vi "lp-server-events.vi"() -> ()   [LabVIEW 2010]
uses:
  socket_type.ctl
  zmq_context.lvclass
  zeromq.lvlib
  zmq_socket.lvclass
panel:
  out "element":string
  out "time (ms)":u32
  in  "stop?":bool
  in  "endpoint":string="tcp://127.0.0.1:5555"
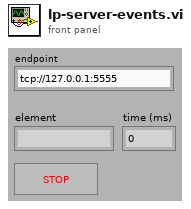
[diagram p1: front panel]
types:
  T1 = typedef "zeromq.lvlib/socket_type.ctl" = enum8{"ZMQ_PAIR", "ZMQ_PUB", "ZMQ_SUB", "ZMQ_REQ", "ZMQ_REP", "ZMQ_DEALER", "ZMQ_ROUTER", "ZMQ_PULL", "ZMQ_PUSH", "ZMQ_XPUB", "ZMQ_XSUB"}
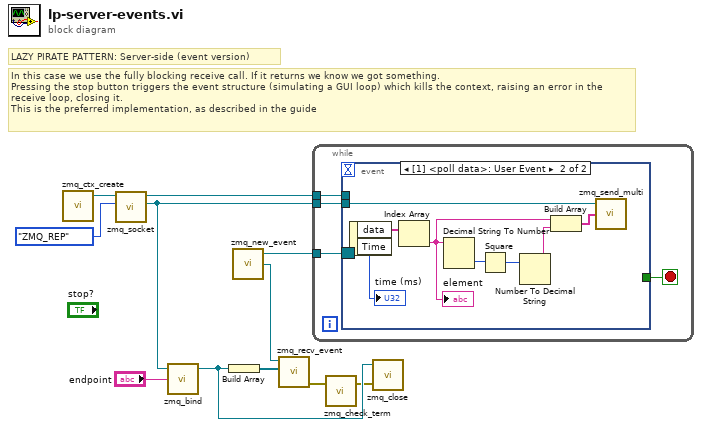
[diagram p0: block diagram]
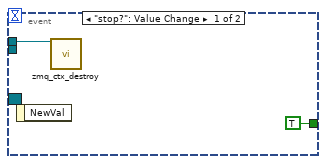
[diagram p2: hidden frame]
diagram:
  # "In this case we use the fully blocking receive call. If it returns we know we got something.\nPressing the stop button triggers the event structure (simulating a GUI loop) which kills the context, raising an error in the receive loop, closing it.\nThis is the preferred implementation, as described in the guide"
  # "LAZY PIRATE PATTERN: Server-side (event version)"
  n1 = call "zmq_ctx_create.vi"() -> ("context out"=w9:refnum<class "zmq_context.lvclass">)  [unwired: 4 in, 1 out]
  n2 = call "zmq_socket.vi"("socket type"=socket_type."ZMQ_REP", "context in"=w9) -> ("socket out"=w4:refnum<class "zmq_socket.lvclass">, "context out"=w8:refnum<class "zmq_context.lvclass">)  [unwired: 3 in, 1 out]
  n3 = call "zmq_bind.vi"("endpoint"="endpoint", "socket in"=w4) -> ("socket out"=w3:refnum<class "zmq_socket.lvclass">)  [unwired: 2 in, 1 out]
  n4 = Build Array(w3) -> (w7:refnum<class "zmq_socket.lvclass">[])
  n5 = call "zmq_new_event.vi"() -> ("user event"=w5:refnum<user-event>, "event ref out"=w6:refnum<event-registration>)  [unwired: 3 in, 1 out]
  n6 = call "zmq_recv_event.vi"("sockets"=w7, "poll event"=w5) -> ("error out"=w2:errorcluster)  [unwired: 4 in, 1 out]
  n7 = while {
    tunnel: w8 -> [w15]
    tunnel: w6 -> [w14]
    tunnel: w4 -> [w13]
    stop <- w12 stop-if-true
    n8 = event shown="[1] <poll data>: User Event" {
      selector: w14 -> [_ _]
      dyn-events: _ -> [_ _]
      timeout: _ -> [_ _]
      tunnel: w15 -> [w17 _]
      tunnel: w13 -> [_ w19]
      tunnel: [TRUE ("NewVal") _] -> w12
      event "stop?": Value Change {
        n9 = event-data() -> ()  [unwired: 1 in, 1 out]
        n10 = call "zmq_ctx_destroy.vi"("context in"=w17) -> ()  [unwired: 4 in, 1 out]
      }
      event User Event {
        n11 = event-data() -> ("data"=w21:string[], "Time"=→"time (ms)":u32)  [unwired: 1 in]
        n12 = Index Array(array=w21) -> (element=w20:string)  [unwired: 1 in]
        "element" <- w20
        n13 = Decimal String To Number(string=w20) -> (number=w22:i32)  [unwired: 2 in, 1 out]
        n14 = Square(x=w22) -> (x^2=w23:i32)
        n15 = Number To Decimal String(number=w23) -> (decimal integer string=w24:string)  [unwired: 1 in]
        n16 = Build Array(w20, w24) -> (w25:string[])
        n17 = call "zmq_send_multi.vi"("parts"=w25, "socket in"=w19) -> ()  [unwired: 2 in, 2 out]
      }
    }
  }
  n18 = call "zmq_check_term.vi"("error in"=w2) -> ("error out"=w1:errorcluster)  [unwired: 1 in, 1 out]
  n19 = call "zmq_close.vi"("error in"=w1, "socket"=w3) -> ()  [unwired: 3 in, 1 out]
